vi "GEA2 Serial Error Bool Enumerator.vi"(5 "Error Enum":T1, 6 "Error In":errorcluster, 8 "Error?":bool=TRUE) -> (0 "Error Out":errorcluster)   [LabVIEW 2014]
uses:
  Type Definitions/GEA2 Serial Dryer Error Enumeration.ctl
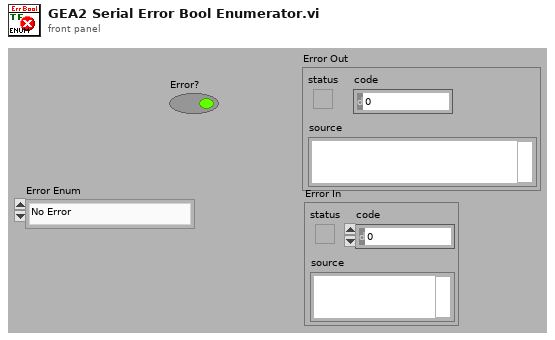
[diagram p1: front panel]
types:
  T1 = typedef "GEA2 Serial Dryer Error Enumeration.ctl" = enum16{"No Error", "GEA2 Send ACK Mismatch", "GEA2 STX", "GEA2 ETX", "GEA2 CRC Mismatch", "GEA2 ReadACK", "RTD In Range Error", "Fail Mean Tank Temp", "No Flow Config Data Found", "Failed Flow During Purge", "Temp During Purge", "Confirm IF Stop Fail", "Init Draw: TC_1 Out of Range", "Flow = 0 During Draw after 20s"}
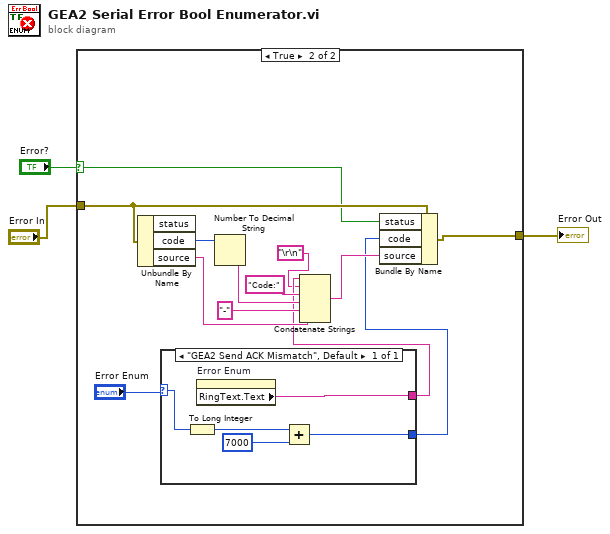
[diagram p0: block diagram]
diagram:
  n1 = case shown="True" "Error?" {
    selector: "Error?" -> [_ w15]
    tunnel: "Error In" -> [w4 w17]
    tunnel: [w4 w12] -> w1
    frame False {
    }
    frame True {
      n2 = Unbundle By Name(w17) -> ("code"=w11:i32, "source"=w14:string)  [unwired: 1 out]
      n3 = case shown="\"GEA2 Send ACK Mismatch\", Default" "Error Enum" {
        selector: "Error Enum" -> [w21]
        tunnel: [w19] -> w7
        tunnel: [w18] -> w6
        frame "GEA2 Send ACK Mismatch", Default {
          n4 = To Long Integer(number=w21) -> (32bit integer=w20:i32)
          n5 = property on="Error Enum" class="Enum (strict)"() -> ("RingText.Text"=w18:string)  [unwired: 2 in, 2 out]
          n6 = Add(x=w20, y=7000) -> (x+y=w19:i32)
        }
      }
      n7 = Number To Decimal String(number=w11) -> (decimal integer string=w10:string)  [unwired: 1 in]
      n8 = Concatenate Strings(w6, "\r\n", "Code:" ("string"), w10, "-" ("string"), w14) -> (w16:string)
      n9 = Bundle By Name(cluster=w17, "status"=w15, "code"=w7, "source"=w16) -> (w12:errorcluster)
    }
  }
  "Error Out" <- w1
